vi "Update Values with Terminals Status.vi"(8 "error in":errorcluster, 10 "values in":dbl[](array[numeric]), 11 "Rx execution unit in":refnum<class "Rx Execution Unit.lvclass">) -> (0 "error out":errorcluster, 2 "values out":dbl[](array[numeric]), 3 "Rx execution unit out":refnum<class "Rx Execution Unit.lvclass">)   [LabVIEW 2020, in "Ballard MIL-STD-1553 Engine.lvlib" / "Implementation.lvlib" / "Rx Execution Unit.lvclass"]
uses:
  Rx Execution Unit.lvclass
  Rx Execution Unit.lvclass/Rx Execution Unit.ctl
  <instrlib>/BTI1553Lib/BTI1553LV.lvlib
  Scripting/Constants.vi
  Scripting/Ballard MIL-STD-1553 Scripting.lvlib
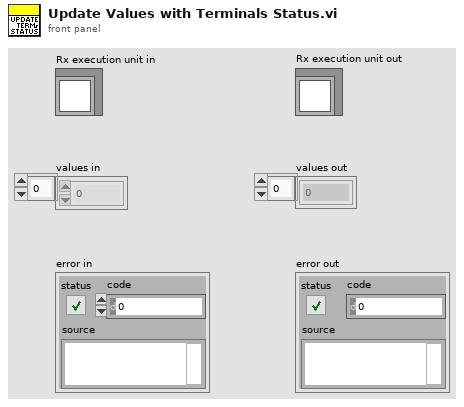
[diagram p1: front panel]
types:
  T1 = typedef "Ballard MIL-STD-1553 Engine.lvlib/Implementation.lvlib/Rx Execution Unit.lvclass/Status Terminal Lookup Data.ctl" = cluster{"value index":i32, "remote terminal handle":u64, "terminal address":u64}
  T2 = typedef "BTI1553LV.lvlib/1553 BC Status.ctl" = u32
  T3 = typedef "BTI1553LV.lvlib/1553 RT Status.ctl" = u32
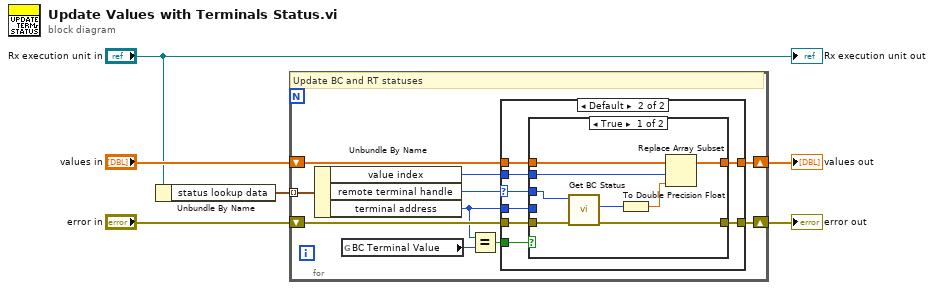
[diagram p0: block diagram]
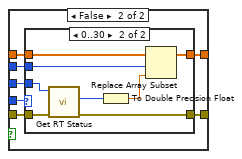
[diagram p3: hidden frame]
diagram:
  n1 = Unbundle By Name("Rx execution unit in") -> ("status lookup data"=w3:T1[])
  n2 = for {
    tunnel: w3 -> [w15] mode=indexing
    shift-right: [w13] -> w5
    shift-left: "error in" -> [w14]
    shift-right: [w10] -> w6
    shift-left: "values in" -> [w11]
    # "Update BC and RT statuses"
    n3 = Unbundle By Name(w15) -> ("value index"=w12:i32, "remote terminal handle"=w16:u64, "terminal address"=w7:u64)
    n4 = global read "Constants.vi" "BC Terminal Value"() -> (w9:u16)
    n5 = Equal?(x=w7, y=w9) -> (x = y?=w8:bool)
    n6 = case shown="Default" w16 {
      selector: w16 -> [_ w26]
      tunnel: w14 -> [w17 w25]
      tunnel: [w17 w24] -> w13
      tunnel: w12 -> [_ w23]
      tunnel: w11 -> [w18 w22]
      tunnel: [w18 w21] -> w10
      tunnel: w8 -> [_ w20]
      tunnel: w7 -> [_ w19]
      frame 0, -1 {
      }
      frame Default {
        n7 = case shown="True" w20 {
          tunnel: w25 -> [w33 w40]
          tunnel: w26 -> [w34 w41]
          tunnel: [w32 w39] -> w24
          tunnel: w23 -> [w30 w38]
          tunnel: w22 -> [w28 w37]
          tunnel: [w27 w36] -> w21
          tunnel: w19 -> [_ w35]
          frame True {
            # "RTs"
            n8 = call <instrlib>:"Get BC Status.vi"("error in (no error)"=w33, "bus controller handle in"=w34) -> ("error out"=w32:errorcluster, "status"=w29:T2)  [unwired: 7 in, 1 out]
            n9 = To Double Precision Float(number=w29) -> (double precision float=w31:dbl)
            n10 = Replace Array Subset(array=w28, new element=w31, index=w30) -> (w27:dbl[])
          }
          frame False {
            # "RTs"
            n11 = case shown="0..30" w35 {
              tunnel: w41 -> [_ w51]
              tunnel: w40 -> [w42 w50]
              tunnel: [w42 w49] -> w39
              tunnel: w38 -> [_ w47]
              tunnel: w37 -> [w43 w45]
              tunnel: [w43 w44] -> w36
              frame Default {
              }
              frame 0..30 {
                n12 = call <instrlib>:"Get RT Status.vi"("error in (no error)"=w50, "remote terminal handle in"=w51) -> ("error out"=w49:errorcluster, "status"=w46:T3)  [unwired: 7 in, 1 out]
                n13 = To Double Precision Float(number=w46) -> (double precision float=w48:dbl)
                n14 = Replace Array Subset(array=w45, new element=w48, index=w47) -> (w44:dbl[])
              }
            }
          }
        }
      }
    }
  }
  "values out" <- w6
  "error out" <- w5
  "Rx execution unit out" <- "Rx execution unit in"
